vi "input.vi"(8 "error in":errorcluster, 10 "data table in":T1, 11 "Modbus Slave runtime in":refnum<class "Modbus Slave runtime.lvclass">) -> (0 "error out":errorcluster, 2 "data table out":T1, 3 "Modbus Slave runtime out":refnum<class "Modbus Slave runtime.lvclass">)   [LabVIEW 2013, in "Modbus Slave runtime.lvclass"]
doc: "Provides an interface for reading data from a module at runtime. While this interface performs no operations, a child should provide an override which may read from any open sessions, references, or interfaces.Platypus Framework 1.0.1.65\nNI Systems Engineering - National Instruments"
uses:
  Modbus Slave runtime.lvclass
  <vilib>/NI/Tag Bus/table/data table.ctl
  Modbus Slave runtime.lvclass/Modbus Slave runtime.ctl
  <vilib>/NI/Modbus Library/API/Slave/Modbus Slave.lvclass
  <vilib>/NI/Tag Bus/table/data table.lvlib
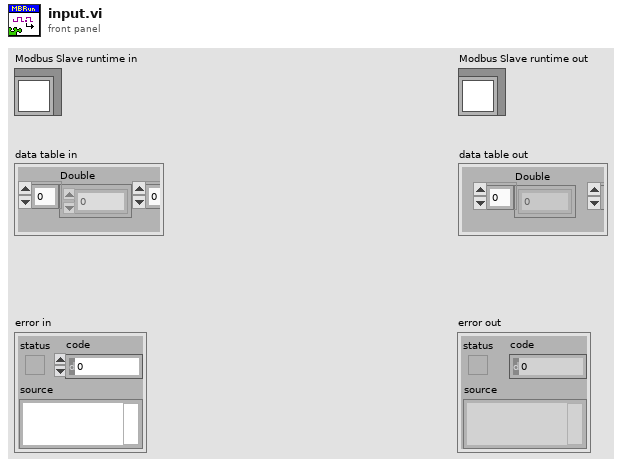
[diagram p1: front panel]
types:
  T1 = typedef "tag bus.lvlib/data table.lvlib/data table.ctl" = cluster{"Double":dbl[], "Single":sgl[], "I64":i64[], "I32":i32[], "I16":i16[], "I8":i8[], "U64":u64[], "U32":u32[], "U16":u16[], "U8":u8[], "Boolean":bool[], "String":string[], "Array of Double":cluster{"DBL Array":dbl[]}[], "Array of Single":cluster{"SGL Array":sgl[]}[], "Array of I64":cluster{"I64 Array":i64[]}[], "Array of I32":cluster{"I32 Array":i32[]}[], "Array of I16":cluster{"I16 Array":i16[]}[], "Array of I8":cluster{"I8 Array":i8[]}[], "Array of U64":cluster{"U64 Array":u64[]}[], "Array of U32":cluster{"U32 Array":u32[]}[], "Array of U16":cluster{"U16 Array":u16[]}[], "Array of U8":cluster{"U8 Array":u8[]}[], "Array of Boolean":cluster{"Boolean Array":bool[]}[], "Array of String":cluster{"String Array":string[]}[]}
  T2 = typedef "Modbus Slave runtime.lvclass/bulk data access.ctl" = cluster{"modbus type":T3, "start":u16, "length":u16, "maps":T4[]}
  T3 = typedef "Modbus Module Channel.lvclass/data bank type.ctl" = enum16{"coils", "discrete inputs", "input registers", "holding registers"}
  T4 = typedef "Modbus Slave runtime.lvclass/data mapping elements.ctl" = cluster{"data type":T5, "data index":i32, "element index":i32, "subindex":i32}
  T5 = typedef "tag bus.lvlib/tag descriptor.lvclass/Data Type.ctl" = enum16{"Double", "Single", "I64", "I32", "I16", "I8", "U64", "U32", "U16", "U8", "Boolean", "String", "Array of Double", "Array of Single", "Array of I64", "Array of I32", "Array of I16", "Array of I8", "Array of U64", "Array of U32", "Array of U16", "Array of U8", "Array of Boolean", "Array of String"}
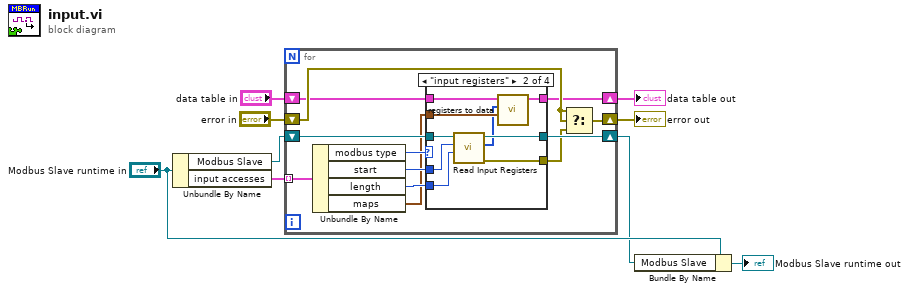
[diagram p0: block diagram]
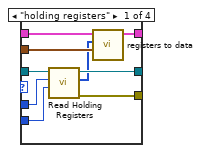
[diagram p2: hidden frame]
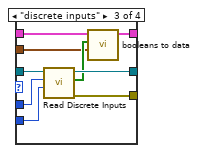
[diagram p3: hidden frame]
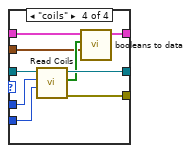
[diagram p4: hidden frame]
diagram:
  n1 = Unbundle By Name("Modbus Slave runtime in") -> ("Modbus Slave"=w7:refnum<class "Modbus Slave.lvclass">, "input accesses"=w3:T2[])
  n2 = for {
    shift-right: [w18] -> w6
    shift-left: w7 -> [w19]
    shift-right: [w20] -> w4
    shift-left: "error in" -> [w21]
    tunnel: w3 -> [w16] mode=indexing
    shift-right: [w11] -> w1
    shift-left: "data table in" -> [w12]
    n3 = Unbundle By Name(w16) -> ("modbus type"=w13:T3, "start"=w14:u16, "length"=w15:u16, "maps"=w10:T4[])
    n4 = case shown="\"input registers\"" w13 {
      tunnel: w19 -> [w28 w37 w46 w55]
      tunnel: [w30 w39 w48 w57] -> w18
      tunnel: [w29 w38 w47 w56] -> w17
      tunnel: w14 -> [w27 w36 w45 w54]
      tunnel: w15 -> [w26 w35 w44 w53]
      tunnel: w12 -> [w25 w34 w43 w51]
      tunnel: [w24 w33 w42 w52] -> w11
      tunnel: w10 -> [w23 w32 w40 w49]
      frame "holding registers" {
        n5 = call-dynamic "Read Holding Registers.vi"("number of inputs"=w26, "starting address"=w27, "Modbus slave in"=w28) -> ("error out"=w29:errorcluster, "register values"=w22:u16[], "Modbus slave out"=w30:refnum<class "Modbus Slave.lvclass">)  [unwired: 6 in]
        n6 = call "registers to data.vi"("specifications"=w23, "registers"=w22, "allocation"=w25) -> ("data table"=w24:T1)  [unwired: 8 in]
      }
      frame "input registers" {
        n7 = call-dynamic "Read Input Registers.vi"("number of inputs"=w35, "starting address"=w36, "Modbus slave in"=w37) -> ("error out"=w38:errorcluster, "register values"=w31:u16[], "Modbus slave out"=w39:refnum<class "Modbus Slave.lvclass">)  [unwired: 6 in]
        n8 = call "registers to data.vi"("specifications"=w32, "registers"=w31, "allocation"=w34) -> ("data table"=w33:T1)  [unwired: 8 in]
      }
      frame "discrete inputs" {
        n9 = call-dynamic "Read Discrete Inputs.vi"("number of inputs"=w44, "starting address"=w45, "Modbus slave in"=w46) -> ("error out"=w47:errorcluster, "discrete inputs"=w41:bool[], "Modbus slave out"=w48:refnum<class "Modbus Slave.lvclass">)  [unwired: 6 in]
        n10 = call "booleans to data.vi"("specifications"=w40, "booleans"=w41, "allocation"=w43) -> ("data table"=w42:T1)  [unwired: 8 in]
      }
      frame "coils" {
        n11 = call-dynamic "Read Coils.vi"("number of inputs"=w53, "starting address"=w54, "Modbus slave in"=w55) -> ("error out"=w56:errorcluster, "coils"=w50:bool[], "Modbus slave out"=w57:refnum<class "Modbus Slave.lvclass">)  [unwired: 6 in]
        n12 = call "booleans to data.vi"("specifications"=w49, "booleans"=w50, "allocation"=w51) -> ("data table"=w52:T1)  [unwired: 8 in]
      }
    }
    n13 = Select(t=w21, s=w21, f=w17) -> (s? t:f=w20:errorcluster)
  }
  "error out" <- w4
  "data table out" <- w1
  n14 = Bundle By Name(cluster="Modbus Slave runtime in", "Modbus Slave"=w6) -> (→"Modbus Slave runtime out":refnum<class "Modbus Slave runtime.lvclass">)
